vi "encoder2kmh.vi"(6 "Gear":enum16{"7", "6", "5", "4", "3", "2", "1"}(ring), 11 "encoderSpeed":sgl) -> (3 "realVelocity":sgl)   [LabVIEW 2016]
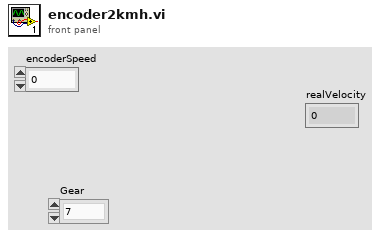
[diagram p1: front panel]
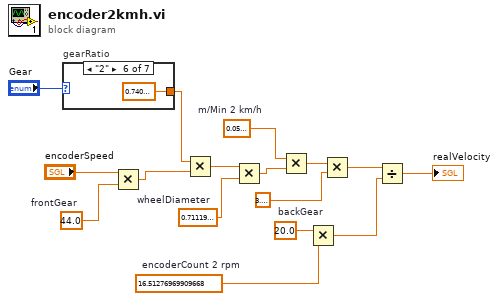
[diagram p0: block diagram]
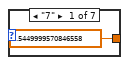
[diagram p2: hidden frame]
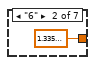
[diagram p3: hidden frame]
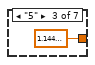
[diagram p4: hidden frame]
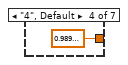
[diagram p5: hidden frame]
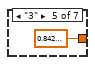
[diagram p6: hidden frame]
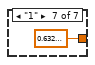
[diagram p7: hidden frame]
diagram:
  w2 = sgl 16.51277  # encoderCount 2 rpm
  w3 = sgl 20.0  # backGear
  w8 = sgl 0.06  # m/Min 2 km/h
  w10 = sgl 0.7112  # wheelDiameter
  w14 = sgl 44.0  # frontGear
  n1 = case "gearRatio" shown="\"2\"" "Gear" {
    tunnel: [sgl 1.545 sgl 1.335 sgl 1.145 sgl 0.989 sgl 0.843 sgl 0.741 sgl 0.632] -> w12
    frame "7" {
    }
    frame "6" {
    }
    frame "5" {
    }
    frame "4", Default {
    }
    frame "3" {
    }
    frame "2" {
    }
    frame "1" {
    }
  }
  n2 = Multiply(x="encoderSpeed", y=w14) -> (x*y=w13:sgl)
  n3 = Multiply(x=w12, y=w13) -> (x*y=w11:sgl)
  n4 = Multiply(x=w11, y=w10) -> (x*y=w9:sgl)
  n5 = Multiply(x=w8, y=w9) -> (x*y=w7:sgl)
  n6 = Multiply(x=w3, y=w2) -> (x*y=w4:sgl)
  n7 = Multiply(x=w7, y=sgl 3.1415927) -> (x*y=w5:sgl)
  n8 = Divide(x=w5, y=w4) -> (x/y=→"realVelocity":sgl)
